vi "Button_Ctrl_Check.vi"(8 "error in (no error)":errorcluster, 11 "Button Ctrl in":T1) -> (0 "error out":errorcluster, 3 "Button Ctrl out":T1)   [LabVIEW 2015]
doc: "Make sure:\n1. Only files are in list, no directories, or empty paths\n2. Only 10 files are in the list\n3. The trigger is appropriate for the number of files"
uses:
  controls/AFCP Setup.ctl
  <userlib>/_OpenG.lib/file/file.llb/File Exists - Scalar__ogtk.vi
  <vilib>/regexp/Match Regular Expression.xnode
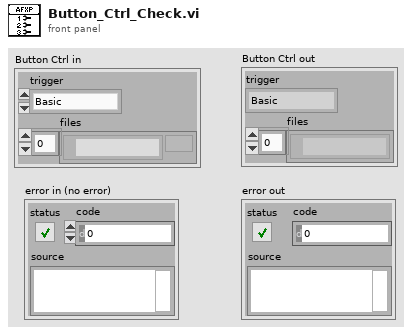
[diagram p1: front panel]
types:
  T1 = typedef "AFCP Setup.ctl" = cluster{"trigger":enum16{"Basic", "Hold-Loop", "Latch-Loop", "Next", "Random", "Disabled"}, "files":path[]}
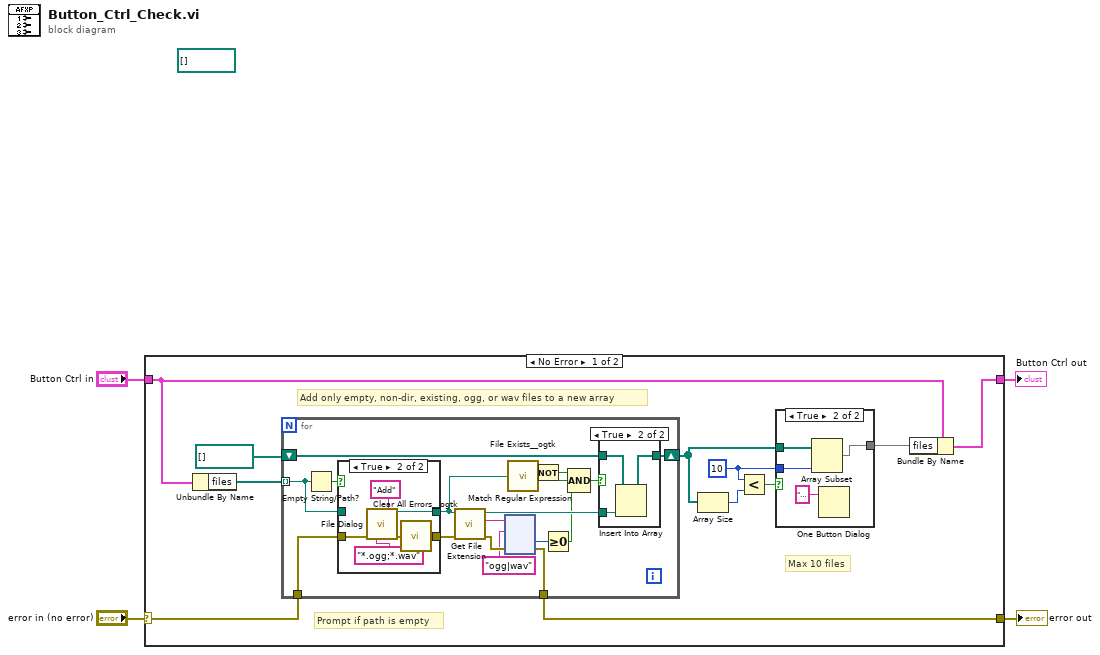
[diagram p0: block diagram]
diagram:
  (unwired) path[] [] ("Sound Files")
  n1 = case shown="No Error" "error in (no error)" {
    selector: "error in (no error)" -> [w5 w165]
    tunnel: [w6 w165] -> w2
    tunnel: [w15 w166] -> w3
    tunnel: "Button Ctrl in" -> [w14 w166]
    frame No Error {
      w10 = 10 ("y")
      # "Add only empty, non-dir, existing, ogg, or wav files to a new array"
      # "Prompt if path is empty"
      # "Max 10 files"
      n2 = Unbundle By Name(w14) -> ("files"=w9:path[])
      n3 = for {
        tunnel: w9 -> [w17] mode=indexing
        shift-right: [w32] -> w8
        shift-left: path[] [] ("Sound Files") -> [w33]
        tunnel: [w28] -> w6
        tunnel: w5 -> [w19]
        n4 = Empty String/Path?(string/path=w17) -> (empty?=w18:bool)
        n5 = case shown="True" w18 {
          tunnel: w19 -> [w34 w41]
          tunnel: w17 -> [w35 _]
          tunnel: [w35 w40] -> w16
          tunnel: [w34 w36] -> w20
          frame False {
            # "not empty"
          }
          frame True {
            # "Path is empty"
            n6 = call "File Dialog"("button label"="Add", "error in"=w41, "pattern (all files)"="*.ogg;*.wav") -> ("selected path"=w40:path, "error out"=w39:errorcluster)  [unwired: 9 in, 2 out]
            n7 = call <userlib>:"Clear All Errors__ogtk.vi"("Error In"=w39) -> ("Error Out"=w36:errorcluster)  [unwired: 3 in]
          }
        }
        n8 = call <vilib>:"Get File Extension.vi"("error in (no error)"=w20, "file"=w16) -> ("error out"=w30:errorcluster, "lowercase file extension"=w26:string, "dup file"=w31:path)  [unwired: 5 in, 2 out]
        n9 = xnode "Match Regular Expression"("input string"=w26, "regular expression"="ogg|wav" ("pattern"), "error in"=w30) -> ("offset past match"=w27:i32, "error out"=w28:errorcluster)  [unwired: 3 in, 3 out]
        n10 = call-poly <userlib>:"File Exists__ogtk.vi"("file path"=w16) -> ("is directory"=w25:bool, "exists"=w23:bool)  [unwired: 6 in]
        n11 = Not(x=w25) -> (.not. x?=w22:bool)
        n12 = Greater Or Equal To 0?(x=w27) -> (x >= 0?=w24:bool)
        n13 = Compound Arithmetic op=AND(w22, w23, w24) -> (w21:bool)
        n14 = case shown="True" w21 {
          tunnel: w33 -> [w156 w159]
          tunnel: [w156 w158] -> w32
          tunnel: w31 -> [_ w157]
          frame False {
            # "None"
          }
          frame True {
            # "Add"
            n15 = Insert Into Array(array=w159, new element=w157) -> (w158:path[])  [unwired: 1 in]
          }
        }
      }
      n16 = Array Size(array=w8) -> (size(s)=w11:i32)
      n17 = Less?(x=w10, y=w11) -> (x < y?=w13:bool)
      n18 = case shown="True" w13 {
        tunnel: w8 -> [w160 w163]
        tunnel: w10 -> [_ w161]
        tunnel: [w160 w162] -> w12
        frame False {
          # "10 or less"
        }
        frame True {
          # "Max 10 files"
          n19 = Array Subset(array=w163, length=w161) -> (w162:path[])  [unwired: 1 in]
          n20 = One Button Dialog(message="Warning: Each button can use a maximum of 10 files!\nUsing only first 10 files...") -> ()  [unwired: 1 in, 1 out]
        }
      }
      n21 = Bundle By Name(cluster=w14, "files"=w12) -> (w15:T1)
    }
    frame Error {
    }
  }
  "error out" <- w2
  "Button Ctrl out" <- w3
